vi "5668 Truncate Spectrum.vi"(10 "Power Spectrum / PSD (dBm)":cluster{"f0":dbl, "df":dbl, "magnitude":dbl[]}, 11 "y":dbl) -> (2 "Array":dbl[](array[numeric]), 3 "df":dbl)   [LabVIEW 2017]
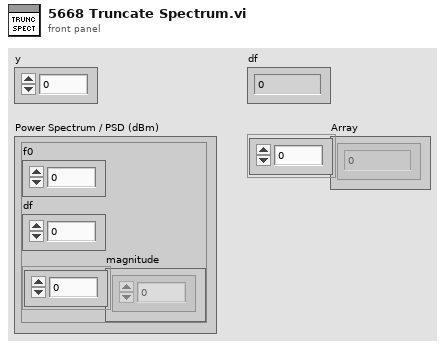
[diagram p1: front panel]
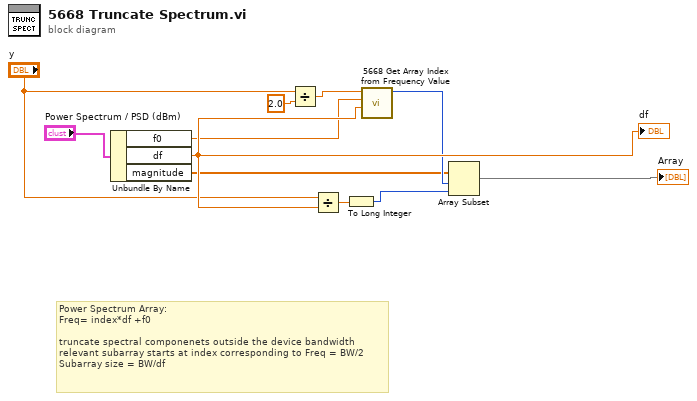
[diagram p0: block diagram]
diagram:
  # "Power Spectrum Array:\nFreq= index*df +f0\n\ntruncate spectral componenets outside the device bandwidth\nrelevant subarray starts at index corresponding to Freq = BW/2\nSubarray size = BW/df"
  n1 = Unbundle By Name("Power Spectrum / PSD (dBm)") -> ("f0"=w5:dbl, "df"=w11:dbl, "magnitude"=w4:dbl[])
  "df" <- w11
  n2 = Divide(x="y", y=2.0) -> (x/y=w2:dbl)
  n3 = Divide(x="y", y=w11) -> (x/y=w8:dbl)
  n4 = To Long Integer(number=w8) -> (32bit integer=w9:i32)
  n5 = call "5668 Get Array Index from Frequency Value.vi"("df"=w11, "f0"=w5, "Numeric Control in"=w2) -> ("Numeric Control out"=w6:i32)  [unwired: 8 in]
  n6 = Array Subset(array=w4, index=w6, length=w9) -> (→"Array":dbl[])
